vi "Cambia file taratura.vi"(10 "FILE ATTUALE":string) -> (1 "NEW FILE":string, 2 "COEFF":T1, 3 "CANCELLED?":bool=TRUE)   [LabVIEW 2019]
uses:
  <vilib>/addons/database/_DB Variant To Data/Database Variant To Data.xnode
  <vilib>/addons/database/NI_Database_API.lvlib
panel:
  in  "OK Button":bool
  in  "Cancel Button":bool
  in  "FILTRO FILE TARATURA MOTORE":T2(radio)
  in  "FILE TARATURA":string(combo)
  # "SELEZIONA NUOVO FILE"
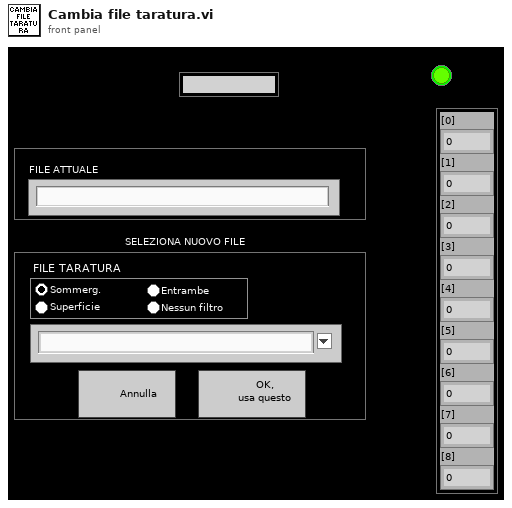
[diagram p1: front panel]
types:
  T1 = cluster{"[0]":dbl, "[1]":dbl, "[2]":dbl, "[3]":dbl, "[4]":dbl, "[5]":dbl, "[6]":dbl, "[7]":dbl, "[8]":dbl}
  T2 = enum32{"Sommergibile", "Superficie", "Entrambe", "Nessun filtro"}
  T3 = typedef "NI_Database_API.lvlib/Conn ObjectReference.ctl" = refnum<k1>
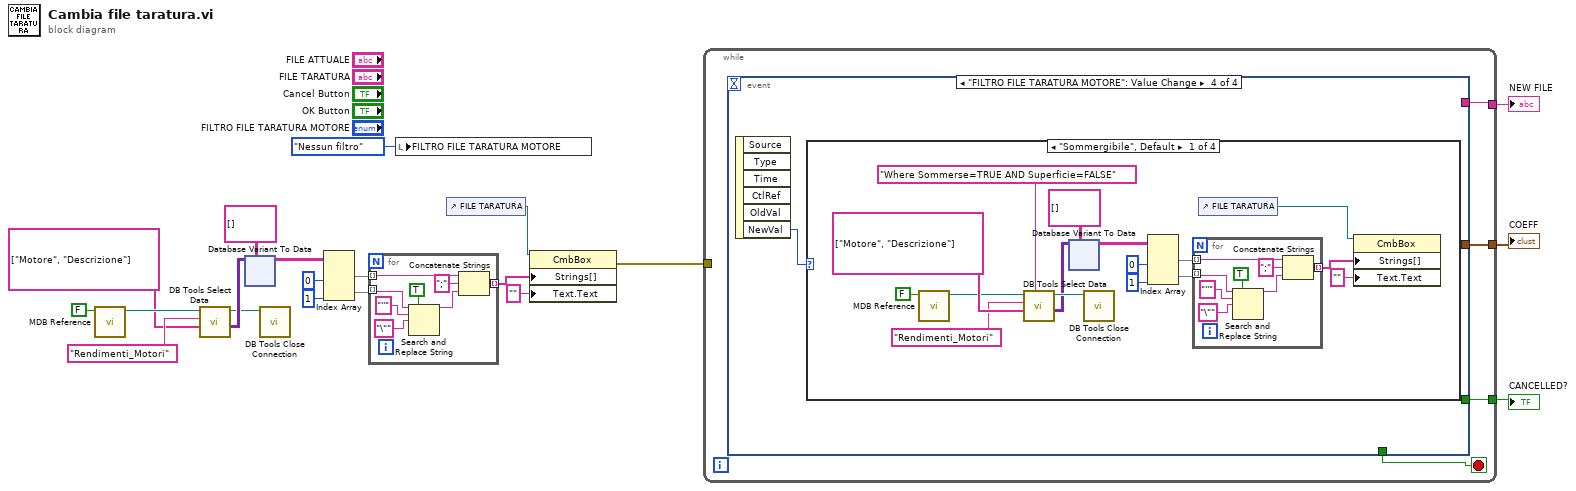
[diagram p0: block diagram]
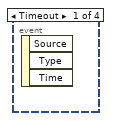
[diagram p2: hidden frame]
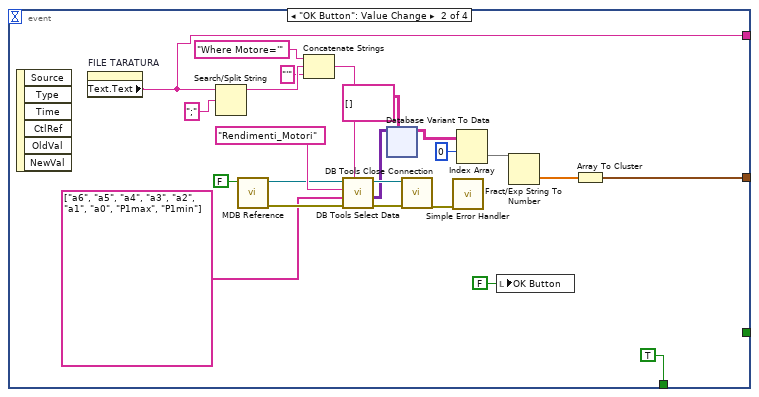
[diagram p3: hidden frame]
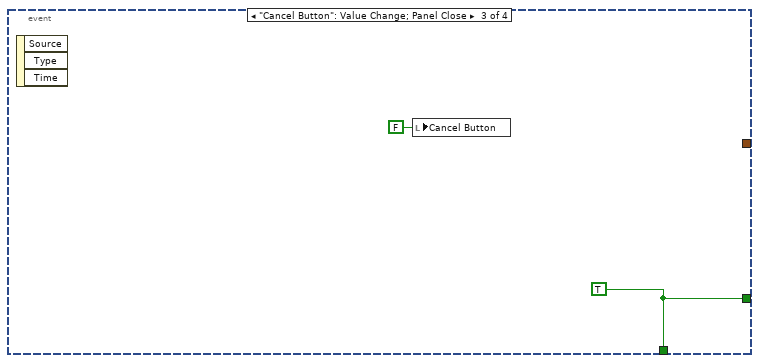
[diagram p4: hidden frame]
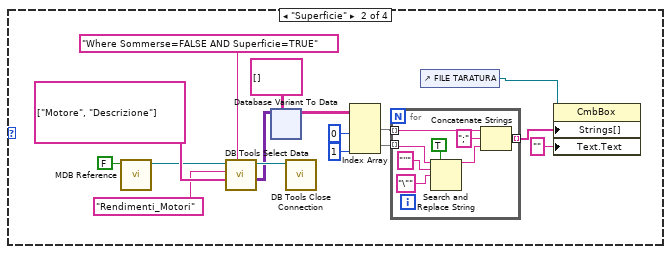
[diagram p5: hidden frame]
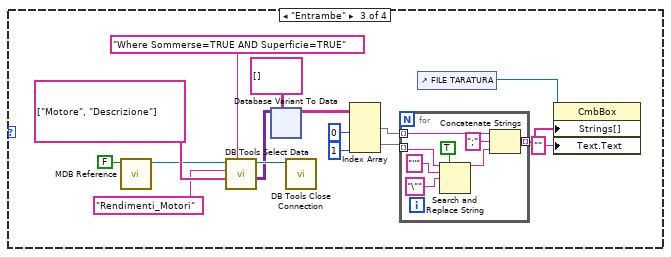
[diagram p6: hidden frame]
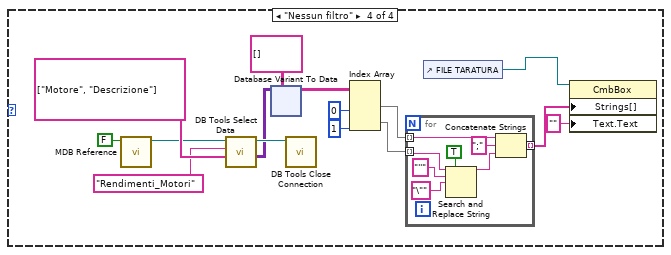
[diagram p7: hidden frame]
diagram:
  n1 = call "MDB Reference.vi"("Collaudi T/motori F"=FALSE ("NM?")) -> ("Refnum out"=w13:T3)  [unwired: 8 in, 2 out]
  n2 = call <vilib>:"DB Tools Select Data.vi"("columns"=string[] ["Motore", "Descrizione"], "table"="Rendimenti_Motori", "connection reference"=w13) -> ("data"=w14:variant[][], "connection reference out"=w8:T3)  [unwired: 3 in, 1 out]
  n3 = xnode "Database Variant To Data"("database variant"=w14, "type"=string[][] [] ("Item Names")) -> ("data"=w10:string[][])  [unwired: 1 in, 1 out]
  n4 = call <vilib>:"DB Tools Close Connection.vi"("connection reference"=w8) -> ()  [unwired: 6 in, 1 out]
  n5 = Index Array(array=w10, index (col) #1=0 ("disabled index (col)"), index (col) #2=1 ("index (col)")) -> (element #1=w17:string[], element #2=w18:string[])  [unwired: 2 in]
  n6 = for {
    tunnel: w17 -> [w28] mode=indexing
    tunnel: w18 -> [w25] mode=indexing
    tunnel: [w26] -> w19 mode=indexing
    n7 = Search and Replace String(replace all?=TRUE ("replace all? (F)"), input string=w25, search string="''" ("substring (\"\")"), replace string="\"" ("replace string (\"\")")) -> (result string=w22:string)  [unwired: 4 in, 3 out]
    n8 = Concatenate Strings(w28, ";" ("string"), w22) -> (w26:string)
  }
  n9 = local write "FILTRO FILE TARATURA MOTORE"(T2."Nessun filtro" ("FILTRO FILE TARATURA MOTORE")) -> ()
  n10 = control-ref of="FILE TARATURA"() -> (w6:refnum<vi>)
  n11 = property class="CmbBox"(reference=w6, "Strings[]"=w19, "Text.Text"="") -> (error out=w4:errorcluster)  [unwired: 1 in, 1 out]
  n12 = while {
    tunnel: w4 -> [_]
    tunnel: [w32] -> w3
    tunnel: [w30] -> w2
    tunnel: [w29] -> w1
    stop <- w31 stop-if-true
    n13 = event shown="[3] \"FILTRO FILE TARATURA MOTORE\": Value Change" {
      selector: _ -> [_ _ _ _]
      dyn-events: _ -> [_ _ _ _]
      timeout: _ -> [_ _ _ _]
      tunnel: [_ w36 _ _] -> w32
      tunnel: [_ TRUE w101 _] -> w31
      tunnel: [_ _ w101 _] -> w30
      tunnel: [_ w33 _ _] -> w29
      event Timeout {
        n14 = event-data() -> ()  [unwired: 1 in, 3 out]
      }
      event "OK Button": Value Change {
        n15 = event-data() -> ()  [unwired: 1 in, 6 out]
        n16 = property on="FILE TARATURA" class="CmbBox"() -> ("Text.Text"=w33:string)  [unwired: 2 in, 2 out]
        n17 = Search/Split String(string=w33, search string/char (-)=";") -> (substring before match=w55:string)  [unwired: 1 in, 2 out]
        n18 = call "MDB Reference.vi"("Collaudi T/motori F"=FALSE ("NM?")) -> ("error out"=w51:errorcluster, "Refnum out"=w40:T3)  [unwired: 8 in, 1 out]
        n19 = Concatenate Strings("Where Motore='" ("condition"), w55, "'" ("string")) -> (w45:string)
        n20 = call <vilib>:"DB Tools Select Data.vi"("condition"=w45, "error in (no error)"=w51, "columns"=string[] ["a6", "a5", "a4", "a3", "a2", "a1", "a0", "P1max", "P1min"], "table"="Rendimenti_Motori", "connection reference"=w40) -> ("error out"=w52:errorcluster, "data"=w39:variant[][], "connection reference out"=w43:T3)  [unwired: 1 in]
        n21 = xnode "Database Variant To Data"("database variant"=w39, "type"=string[][] [] ("Item Names")) -> ("data"=w47:string[][])  [unwired: 1 in, 1 out]
        n22 = call <vilib>:"DB Tools Close Connection.vi"("error in (no error)"=w52, "connection reference"=w43) -> ("error out"=w53:errorcluster)  [unwired: 5 in]
        n23 = call <vilib>:"Simple Error Handler.vi"("error in (no error)"=w53) -> ()  [unwired: 4 in, 5 out]
        n24 = Index Array(array=w47, index (row)=0) -> (element=w49:string[])  [unwired: 1 in]
        n25 = local write "OK Button"(FALSE ("OK Button")) -> ()
        n26 = Fract/Exp String To Number(string=w49) -> (number=w50:dbl[])  [unwired: 3 in, 1 out]
        n27 = Array To Cluster(array=w50) -> (cluster=w36:T1)
      }
      event "Cancel Button": Value Change; Panel Close {
        w101 = TRUE
        n28 = event-data() -> ()  [unwired: 1 in, 3 out]
        n29 = local write "Cancel Button"(FALSE ("Cancel Button")) -> ()
      }
      event "FILTRO FILE TARATURA MOTORE": Value Change {
        n30 = event-data() -> ("NewVal"=w102:T2)  [unwired: 1 in, 5 out]
        n31 = case shown="\"Sommergibile\", Default" w102 {
          frame "Sommergibile", Default {
            n32 = call "MDB Reference.vi"("Collaudi T/motori F"=FALSE ("NM?")) -> ("Refnum out"=w112:T3)  [unwired: 8 in, 2 out]
            n33 = call <vilib>:"DB Tools Select Data.vi"("condition"="Where Sommerse=TRUE AND Superficie=FALSE", "columns"=string[] ["Motore", "Descrizione"], "table"="Rendimenti_Motori", "connection reference"=w112) -> ("data"=w111:variant[][], "connection reference out"=w117:T3)  [unwired: 2 in, 1 out]
            n34 = xnode "Database Variant To Data"("database variant"=w111, "type"=string[][] [] ("Item Names")) -> ("data"=w115:string[][])  [unwired: 1 in, 1 out]
            n35 = call <vilib>:"DB Tools Close Connection.vi"("connection reference"=w117) -> ()  [unwired: 6 in, 1 out]
            n36 = Index Array(array=w115, index (col) #1=0 ("disabled index (col)"), index (col) #2=1 ("index (col)")) -> (element #1=w107:string[], element #2=w106:string[])  [unwired: 2 in]
            n37 = for {
              tunnel: w107 -> [w126] mode=indexing
              tunnel: w106 -> [w123] mode=indexing
              tunnel: [w124] -> w105 mode=indexing
              n38 = Search and Replace String(replace all?=TRUE ("replace all? (F)"), input string=w123, search string="''" ("substring (\"\")"), replace string="\"" ("replace string (\"\")")) -> (result string=w120:string)  [unwired: 4 in, 3 out]
              n39 = Concatenate Strings(w126, ";" ("string"), w120) -> (w124:string)
            }
            n40 = control-ref of="FILE TARATURA"() -> (w103:refnum<vi>)
            n41 = property class="CmbBox"(reference=w103, "Strings[]"=w105, "Text.Text"="") -> ()  [unwired: 1 in, 2 out]
          }
          frame "Superficie" {
            n42 = call "MDB Reference.vi"("Collaudi T/motori F"=FALSE ("NM?")) -> ("Refnum out"=w180:T3)  [unwired: 8 in, 2 out]
            n43 = call <vilib>:"DB Tools Select Data.vi"("condition"="Where Sommerse=FALSE AND Superficie=TRUE", "columns"=string[] ["Motore", "Descrizione"], "table"="Rendimenti_Motori", "connection reference"=w180) -> ("data"=w179:variant[][], "connection reference out"=w185:T3)  [unwired: 2 in, 1 out]
            n44 = xnode "Database Variant To Data"("database variant"=w179, "type"=string[][] [] ("Item Names")) -> ("data"=w183:string[][])  [unwired: 1 in, 1 out]
            n45 = call <vilib>:"DB Tools Close Connection.vi"("connection reference"=w185) -> ()  [unwired: 6 in, 1 out]
            n46 = Index Array(array=w183, index (col) #1=0 ("disabled index (col)"), index (col) #2=1 ("index (col)")) -> (element #1=w175:string[], element #2=w174:string[])  [unwired: 2 in]
            n47 = for {
              tunnel: w175 -> [w194] mode=indexing
              tunnel: w174 -> [w191] mode=indexing
              tunnel: [w192] -> w173 mode=indexing
              n48 = Search and Replace String(replace all?=TRUE ("replace all? (F)"), input string=w191, search string="''" ("substring (\"\")"), replace string="\"" ("replace string (\"\")")) -> (result string=w188:string)  [unwired: 4 in, 3 out]
              n49 = Concatenate Strings(w194, ";" ("string"), w188) -> (w192:string)
            }
            n50 = control-ref of="FILE TARATURA"() -> (w171:refnum<vi>)
            n51 = property class="CmbBox"(reference=w171, "Strings[]"=w173, "Text.Text"="") -> ()  [unwired: 1 in, 2 out]
          }
          frame "Entrambe" {
            n52 = call "MDB Reference.vi"("Collaudi T/motori F"=FALSE ("NM?")) -> ("Refnum out"=w248:T3)  [unwired: 8 in, 2 out]
            n53 = call <vilib>:"DB Tools Select Data.vi"("condition"="Where Sommerse=TRUE AND Superficie=TRUE", "columns"=string[] ["Motore", "Descrizione"], "table"="Rendimenti_Motori", "connection reference"=w248) -> ("data"=w247:variant[][], "connection reference out"=w253:T3)  [unwired: 2 in, 1 out]
            n54 = xnode "Database Variant To Data"("database variant"=w247, "type"=string[][] [] ("Item Names")) -> ("data"=w251:string[][])  [unwired: 1 in, 1 out]
            n55 = call <vilib>:"DB Tools Close Connection.vi"("connection reference"=w253) -> ()  [unwired: 6 in, 1 out]
            n56 = Index Array(array=w251, index (col) #1=0 ("disabled index (col)"), index (col) #2=1 ("index (col)")) -> (element #1=w243:string[], element #2=w242:string[])  [unwired: 2 in]
            n57 = for {
              tunnel: w243 -> [w262] mode=indexing
              tunnel: w242 -> [w259] mode=indexing
              tunnel: [w260] -> w241 mode=indexing
              n58 = Search and Replace String(replace all?=TRUE ("replace all? (F)"), input string=w259, search string="''" ("substring (\"\")"), replace string="\"" ("replace string (\"\")")) -> (result string=w256:string)  [unwired: 4 in, 3 out]
              n59 = Concatenate Strings(w262, ";" ("string"), w256) -> (w260:string)
            }
            n60 = control-ref of="FILE TARATURA"() -> (w239:refnum<vi>)
            n61 = property class="CmbBox"(reference=w239, "Strings[]"=w241, "Text.Text"="") -> ()  [unwired: 1 in, 2 out]
          }
          frame "Nessun filtro" {
            n62 = call "MDB Reference.vi"("Collaudi T/motori F"=FALSE ("NM?")) -> ("Refnum out"=w312:T3)  [unwired: 8 in, 2 out]
            n63 = call <vilib>:"DB Tools Select Data.vi"("columns"=string[] ["Motore", "Descrizione"], "table"="Rendimenti_Motori", "connection reference"=w312) -> ("data"=w311:variant[][], "connection reference out"=w317:T3)  [unwired: 3 in, 1 out]
            n64 = xnode "Database Variant To Data"("database variant"=w311, "type"=string[][] [] ("Item Names")) -> ("data"=w315:string[][])  [unwired: 1 in, 1 out]
            n65 = call <vilib>:"DB Tools Close Connection.vi"("connection reference"=w317) -> ()  [unwired: 6 in, 1 out]
            n66 = Index Array(array=w315, index (col) #1=0 ("disabled index (col)"), index (col) #2=1 ("index (col)")) -> (element #1=w319:string[], element #2=w320:string[])  [unwired: 2 in]
            n67 = for {
              tunnel: w319 -> [w329] mode=indexing
              tunnel: w320 -> [w326] mode=indexing
              tunnel: [w327] -> w321 mode=indexing
              n68 = Search and Replace String(replace all?=TRUE ("replace all? (F)"), input string=w326, search string="''" ("substring (\"\")"), replace string="\"" ("replace string (\"\")")) -> (result string=w323:string)  [unwired: 4 in, 3 out]
              n69 = Concatenate Strings(w329, ";" ("string"), w323) -> (w327:string)
            }
            n70 = control-ref of="FILE TARATURA"() -> (w307:refnum<vi>)
            n71 = property class="CmbBox"(reference=w307, "Strings[]"=w321, "Text.Text"="") -> ()  [unwired: 1 in, 2 out]
          }
        }
      }
    }
  }
  "COEFF" <- w3
  "CANCELLED?" <- w2
  "NEW FILE" <- w1
